vi "Overall_Test.vi"() -> ()   [LabVIEW 2020]
uses:
  <vilib>/DAQmx/read.llb/DAQmx Read (Digital Bool 1Line 1Point).vi
  <vilib>/DAQmx/read.llb/DAQmx Read (Analog 1D Wfm NChan NSamp).vi
  <vilib>/Utility/file.llb/Read Delimited Spreadsheet (DBL).vi
  <vilib>/DAQmx/create/channels.llb/DAQmx Create Channel (AI-Acceleration-Accelerometer).vi
  <vilib>/DAQmx/configure/timing.llb/DAQmx Timing (Sample Clock).vi
  <vilib>/DAQmx/create/channels.llb/DAQmx Create Channel (DI-Digital Input).vi
  <vilib>/DAQmx/miscellaneous.llb/DAQmx Fill In Error Info.vi
  <vilib>/express/express analysis/Spectral/Block/exnSpectralBlock spectral measurements RMS poly.vi
  <vilib>/express/express analysis/Spectral/Block/exnSpectralBlock spectral measurements RMS array WFM.vi
  <vilib>/express/express analysis/Spectral/Block/exnSpectralBlock spectral measurements RMS WFM.vi
  <vilib>/express/express analysis/Spectral/XNode/ExpressSpectralMeasurementsBlockNode.xnode
  <resource>/objmgr/daqmx.rc
panel:
  out "data 3":cluster{"f0":dbl, "df":dbl, "magnitude":dbl[]}(graph) caption="Excitation waveform FFT"
  out "Waveform size(s)":i32
  out "Trigger":bool
  in  "stop":bool
  out "data":waveform(dbl)[](graph) caption="Acceleration"
  out "data 2":cluster{"f0":dbl, "df":dbl, "magnitude":dbl[]}[](graph) caption="Acceleration FFT"
  in  "Scale":dbl
  out "Excitation waveform":waveform(dbl)(graph)
  in  "file to run":path=path "C:/Users/Puja/Desktop/Labview(PC)/Input_Signal/Sine_wave_data_without_time/data1_w1_NT_1per.txt"
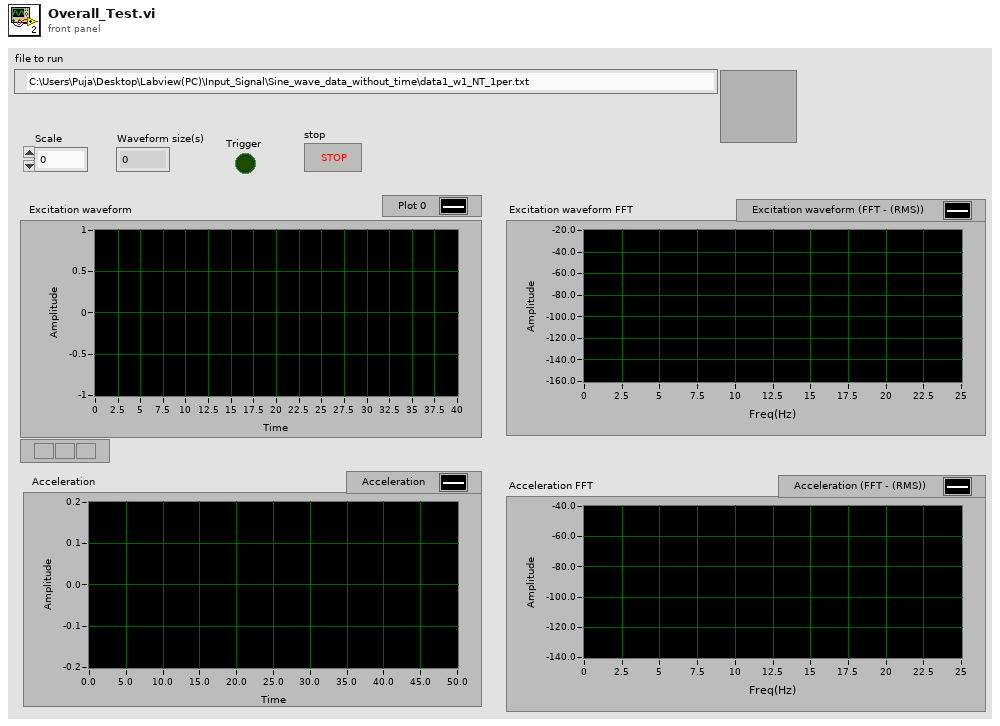
[diagram p1: front panel]
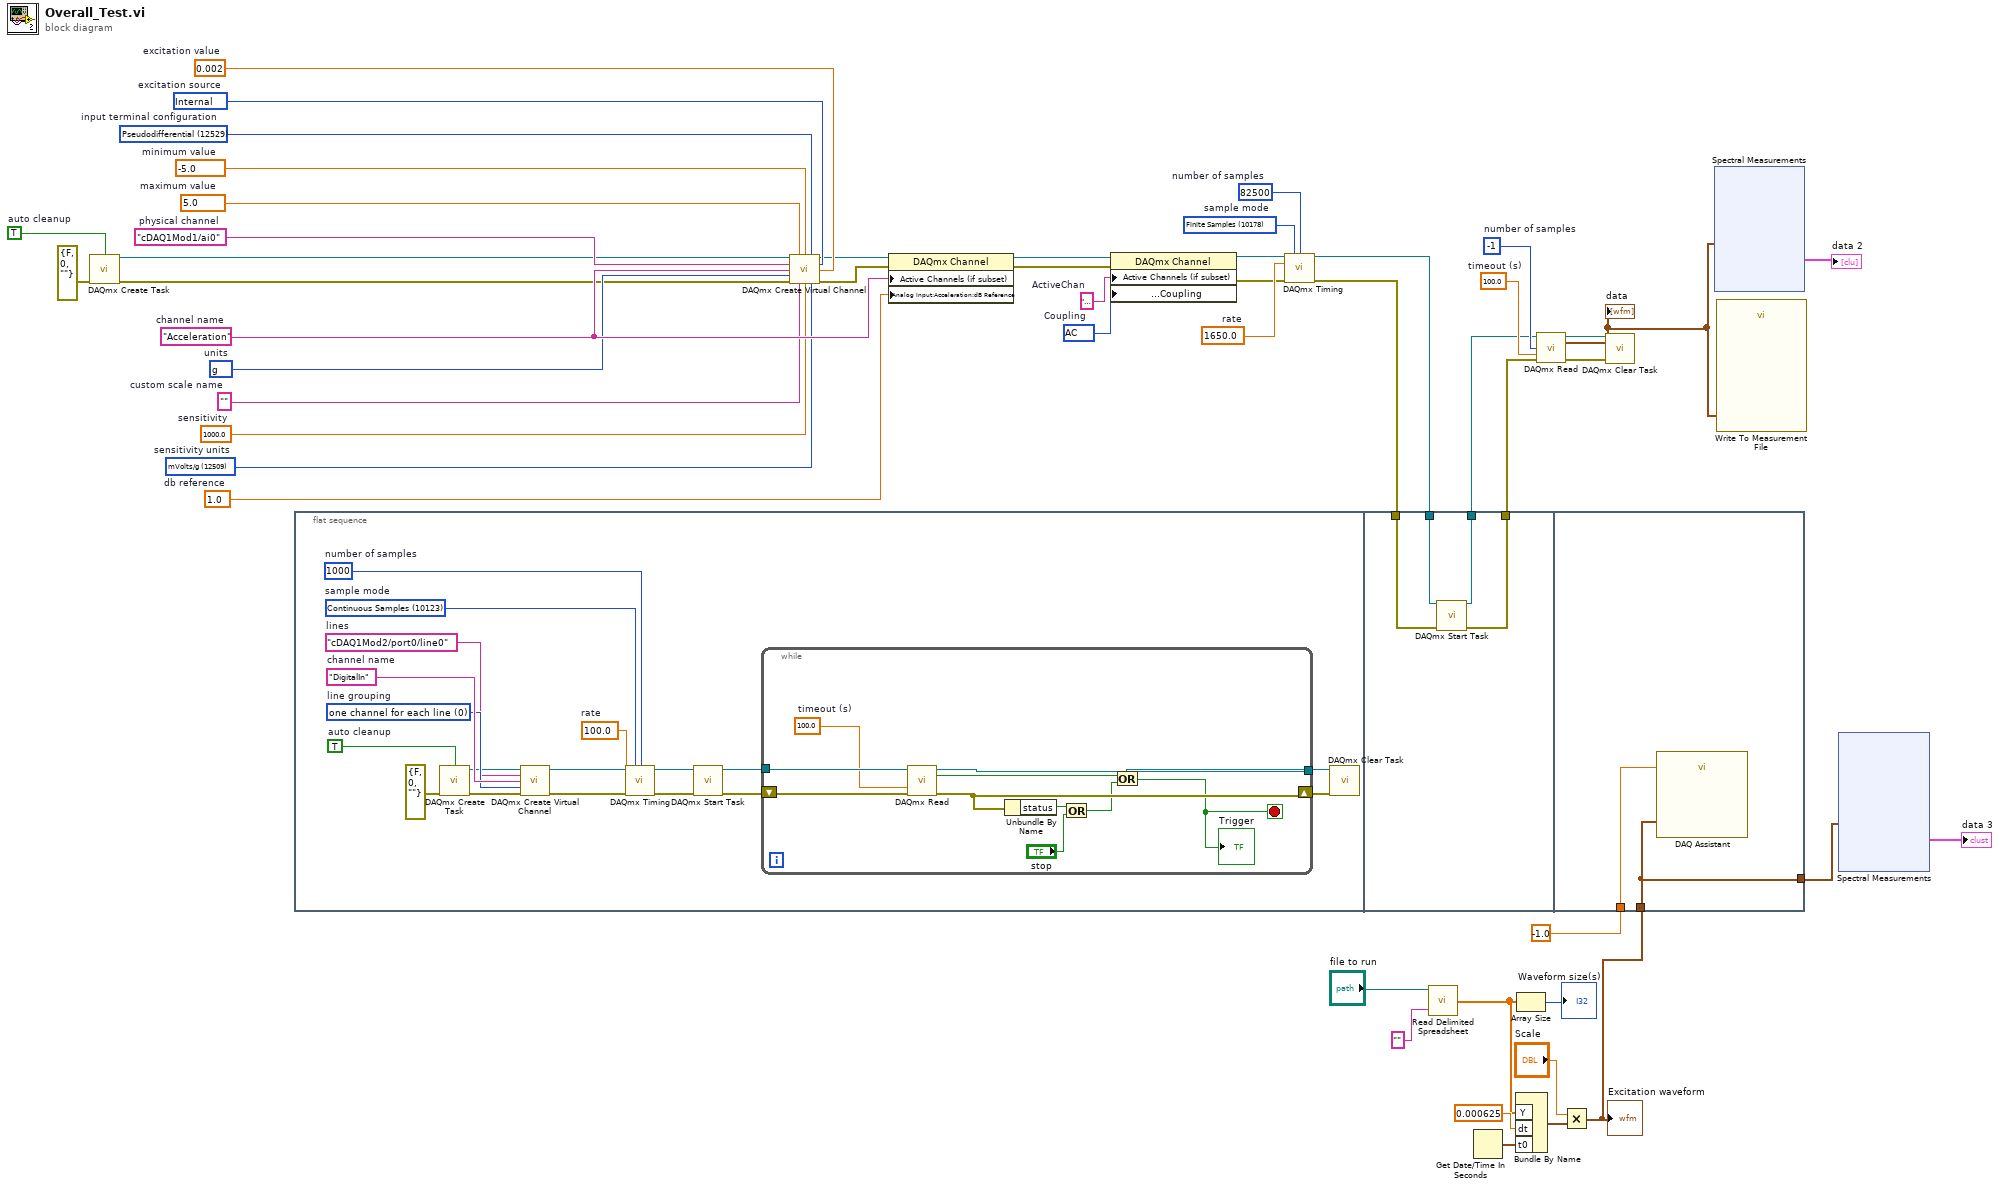
[diagram p0: block diagram]
diagram:
  w38 = 10178 items=["Finite Samples"=10178, "Continuous Samples"=10123, "Hardware Timed Single Point"=12522]  # sample mode
  w37 = 82500  # number of samples
  w36 = 1650.0  # rate
  w32 = 10045 items=["AC"=10045, "DC"=10050, "GND"=10066]  # Coupling
  w31 = "Acceleration"  # ActiveChan
  w29 = 1.0  # db reference
  w26 = 10186 items=["g"=10186, "m/s^2"=12470, "From Custom Scale"=10065]  # units
  w25 = 12529 items=["default"=-1, "RSE"=10083, "NRSE"=10078, "Differential"=10106, "Pseudodifferential"=12529]  # input terminal configuration
  w24 = 10200 items=["Internal"=10200, "External"=10167, "None"=10230]  # excitation source
  w23 = 0.002  # excitation value
  w22 = 12509 items=["mVolts/g"=12509, "Volts/g"=12510]  # sensitivity units
  w21 = 1000.0  # sensitivity
  w30 = "Acceleration"  # channel name
  w19 = ""  # custom scale name
  w18 = -5.0  # minimum value
  w17 = 5.0  # maximum value
  w16 = "cDAQ1Mod1/ai0"  # physical channel
  w14 = TRUE  # auto cleanup
  w42 = 100.0  # timeout (s)
  w43 = -1  # number of samples
  n1 = call <vilib>:"DAQmx Create Task.vi"("auto cleanup"=w14, "error in"=errorcluster {"status"=FALSE, "code"=0, "source"=""}) -> ("task out"=w15:refnum<k21>, "error out"=w13:errorcluster)  [unwired: 12 in]
  n2 = flat-sequence {
    tunnel: w12 -> [w81]
    tunnel: w11 -> [w80]
    tunnel: [w79] -> w10
    tunnel: [w78] -> w9
    tunnel: w7 -> [w82]
    tunnel: -1.0 ("timeout (s)") -> [w83]
    tunnel: [w82] -> w2
    frame #0 {
      w60 = 10123 items=["Finite Samples"=10178, "Continuous Samples"=10123, "Hardware Timed Single Point"=12522]  # sample mode
      w59 = 1000  # number of samples
      w58 = 100.0  # rate
      w54 = 0 items=["one channel for each line", "one channel for all lines"]  # line grouping
      w55 = "DigitalIn"  # channel name
      w53 = "cDAQ1Mod2/port0/line0"  # lines
      w51 = TRUE  # auto cleanup
      n3 = call <vilib>:"DAQmx Create Task.vi"("auto cleanup"=w51, "error in"=errorcluster {"status"=FALSE, "code"=0, "source"=""}) -> ("task out"=w52:refnum<k21>, "error out"=w50:errorcluster)  [unwired: 12 in]
      n4 = call-poly <vilib>:"DAQmx Create Virtual Channel.vi"("task in"=w52, "lines"=w53, "name to assign"=w55, "line grouping"=w54, "error in"=w50) -> ("task out"=w57:refnum<k21>, "error out"=w56:errorcluster)  [unwired: 9 in]
      n5 = call-poly <vilib>:"DAQmx Timing.vi"("task/channels in"=w57, "sample mode"=w60, "samples per channel"=w59, "rate"=w58, "error in"=w56) -> ("task out"=w63:refnum<k21>, "error out"=w62:errorcluster)  [unwired: 9 in]
      n6 = call <vilib>:"DAQmx Start Task.vi"("task/channels in"=w63, "error in"=w62) -> ("task out"=w67:refnum<k21>, "error out"=w66:errorcluster)  [unwired: 12 in]
      n7 = while {
        tunnel: w67 -> [w77]
        tunnel: [w75] -> w64
        shift-right: [w73] -> w65
        shift-left: w66 -> [w76]
        stop <- w69 stop-if-true
        w71 = 100.0  # timeout (s)
        n8 = call-poly <vilib>:"DAQmx Read.vi"("task/channels in"=w77, "timeout"=w71, "error in"=w76) -> ("task out"=w75:refnum<k21>, "data"=w68:bool, "error out"=w73:errorcluster)  [unwired: 10 in]
        n9 = Unbundle By Name(w73) -> ("status"=w74:bool)
        n10 = Or(x=w74, y="stop") -> (x .or. y?=w70:bool)
        n11 = Or(x=w68, y=w70) -> (x .or. y?=w69:bool)
        "Trigger" <- w69
      }
      n12 = call <vilib>:"DAQmx Clear Task.vi"("task in"=w64, "error in"=w65) -> ()  [unwired: 13 in, 1 out]
    }
    frame #1 {
      n13 = call <vilib>:"DAQmx Start Task.vi"("task/channels in"=w81, "error in"=w80) -> ("task out"=w79:refnum<k21>, "error out"=w78:errorcluster)  [unwired: 12 in]
    }
    frame #2 {
      n14 = call "DAQ Assistant"("data"=w82, "timeout (s)"=w83) -> ()  [unwired: 16 in, 2 out]
    }
  }
  n15 = call-poly <vilib>:"DAQmx Create Virtual Channel.vi"("task in"=w15, "maximum value"=w17, "minimum value"=w18, "input terminal configuration"=w25, "physical channels"=w16, "current excitation source"=w24, "name to assign"=w30, "current excitation value"=w23, "units"=w26, "error in"=w13, "custom scale name"=w19, "sensitivity"=w21, "sensitivity units"=w22) -> ("task out"=w20:refnum<k21>, "error out"=w27:errorcluster)  [unwired: 1 in]
  n16 = property class="DAQmx Channel"(reference=w20, error in=w27, "Active Channels (if subset)"=w30, "Analog Input:Acceleration:dB Reference"=w29) -> (reference out=w34:refnum<k21>, error out=w28:errorcluster)
  n17 = property class="DAQmx Channel"(reference=w34, error in=w28, "Active Channels (if subset)"=w31, "Analog Input:General Properties:Input Configuration:Coupling"=w32) -> (reference out=w35:refnum<k21>, error out=w33:errorcluster)
  n18 = call-poly <vilib>:"DAQmx Timing.vi"("task/channels in"=w35, "sample mode"=w38, "samples per channel"=w37, "rate"=w36, "error in"=w33) -> ("task out"=w12:refnum<k21>, "error out"=w11:errorcluster)  [unwired: 9 in]
  n19 = call-poly <vilib>:"Read Delimited Spreadsheet.vi"("file path (dialog if empty)"="file to run", "delimiter (\\t)"="") -> ("first row"=w5:dbl[])  [unwired: 8 in, 5 out]
  n20 = Get Date/Time In Seconds() -> (seconds since 1Jan1904=w47:timestamp)
  n21 = Bundle By Name("Y"=w5, "dt"=0.000625, "t0"=w47) -> (w45:waveform(dbl))  [unwired: 1 in]
  n22 = Array Size(array=w5) -> (size(s)=→"Waveform size(s)":i32)
  n23 = call-poly <vilib>:"DAQmx Read.vi"("task/channels in"=w10, "number of samples per channel"=w43, "timeout"=w42, "error in"=w9) -> ("task out"=w40:refnum<k21>, "data"=w8:waveform(dbl)[], "error out"=w41:errorcluster)  [unwired: 9 in]
  "data" <- w8
  n24 = Multiply(x="Scale", y=w45) -> (x*y=w7:waveform(dbl))
  "Excitation waveform" <- w7
  n25 = call <vilib>:"DAQmx Clear Task.vi"("task in"=w40, "error in"=w41) -> ()  [unwired: 13 in, 1 out]
  n26 = xnode "Spectral Measurements"("Signals"=w8) -> ("FFT - (RMS)"=→"data 2":cluster{"f0":dbl, "df":dbl, "magnitude":dbl[]}[])  [unwired: 1 in, 2 out]
  n27 = call "Write To Measurement File"("Signals"=w8) -> ()  [unwired: 16 in, 3 out]
  n28 = xnode "Spectral Measurements"("Signals"=w2) -> ("FFT - (RMS)"=→"data 3":cluster{"f0":dbl, "df":dbl, "magnitude":dbl[]})  [unwired: 1 in, 2 out]
